vi "AI Post Step.vi"(8 "error in (no error)":errorcluster, 9 "AIRead":T1, 10 "Socket No":u16=1, 11 "NI Analog Input in":refnum<class "NI Analog Input.lvclass">) -> (0 "error out":errorcluster, 1 "AnalogRead":dbl[](array[numeric]), 2 "Report Text":string, 3 "NI Analog Input out":refnum<class "NI Analog Input.lvclass">, 4 "Selected Physical Channel":string[](array[string]))   [LabVIEW 2023, in "HardwareAbstractionLayer_LVOOP.lvlib" / "NI Analog Input.lvclass"]
uses:
  NI Analog Input.lvclass
  NI Analog Input.lvclass/NI Analog Input.ctl
  Database/Database.lvclass
  <resource>/objmgr/daqmx.rc
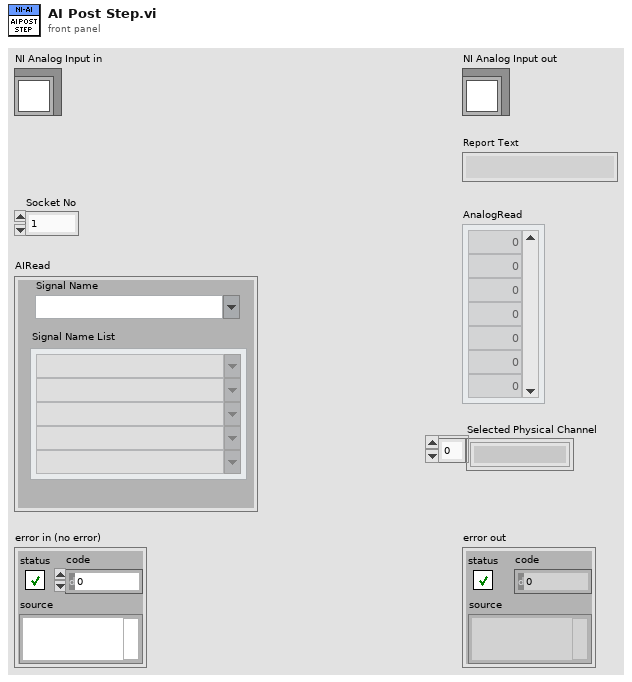
[diagram p1: front panel]
types:
  T1 = cluster{"Signal Name":string, "Signal Name List":string[]}
  T2 = cluster{"table":string, "condition":string, "columns":string[]}
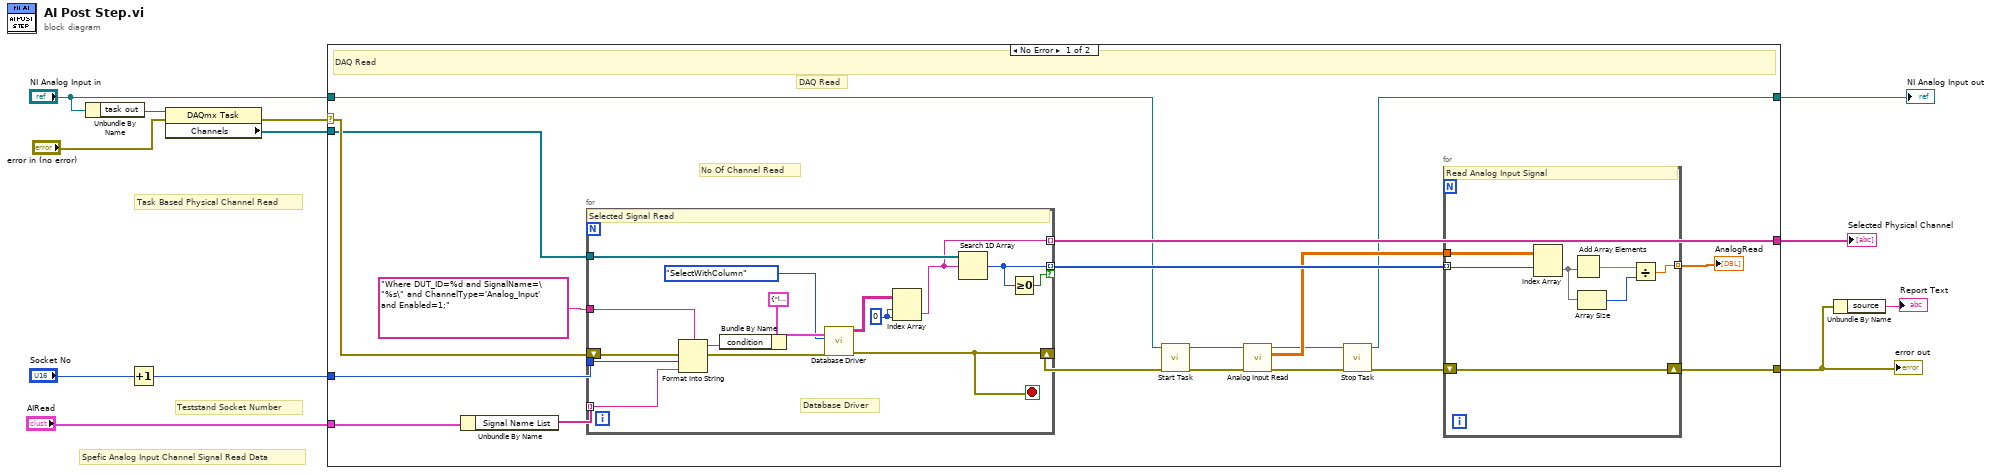
[diagram p0: block diagram]
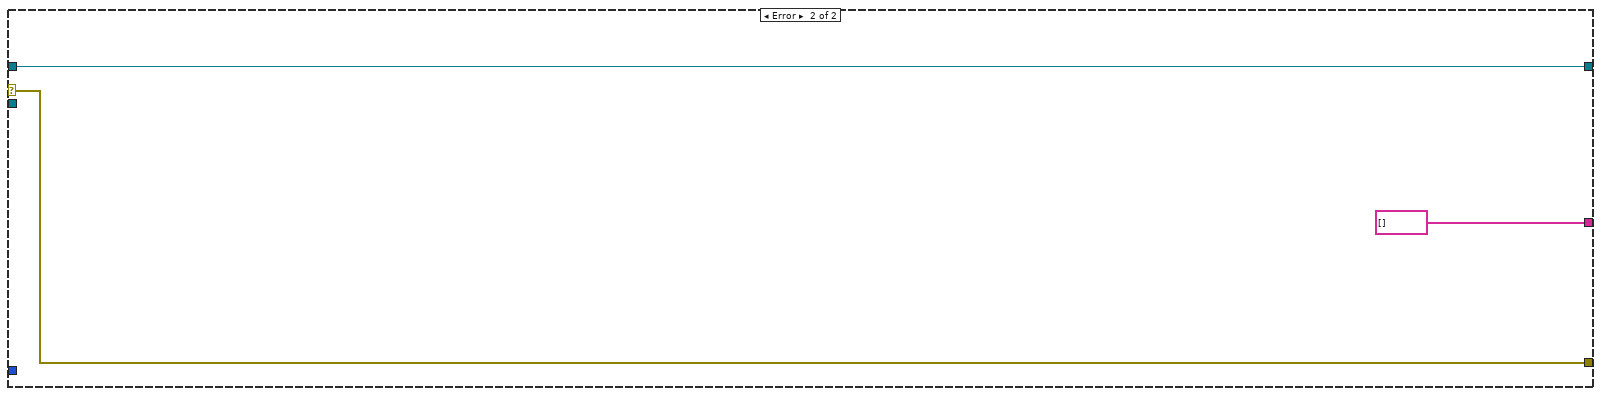
[diagram p2: hidden frame]
diagram:
  # "Teststand Socket Number"
  # "Spefic Analog Input Channel Signal Read Data"
  # "Task Based Physical Channel Read"
  n1 = Unbundle By Name("NI Analog Input in") -> ("task out"=w12:refnum<k21>)
  n2 = Increment(x="Socket No") -> (x+1=w4:u16)
  n3 = property class="DAQmx Task"(reference=w12, error in="error in (no error)") -> (error out=w2:errorcluster, "Channels"=w10:refnum<k21>[])  [unwired: 1 out]
  n4 = case shown="No Error" w2 {
    selector: w2 -> [w25 w56]
    tunnel: [w31 w56] -> w6
    tunnel: "AIRead" -> [w30 _]
    tunnel: w4 -> [w26 _]
    tunnel: w10 -> [w24 _]
    tunnel: "NI Analog Input in" -> [w20 w57]
    tunnel: [w15 w57] -> w7
    tunnel: [w21 string[] []] -> w1
    frame No Error {
      # "No Of Channel Read"
      # "DAQ Read"
      # "DAQ Read"
      n5 = Unbundle By Name(w30) -> ("Signal Name List"=w29:string[])
      n6 = for {
        tunnel: w29 -> [w45] mode=indexing
        tunnel: "Where DUT_ID=%d and SignalName=\"%s\" and ChannelType='Analog_Input' and Enabled=1;" -> [w47]
        tunnel: w26 -> [w46]
        shift-right: [w35] -> w18
        shift-left: w25 -> [w41]
        tunnel: [w37] -> w27 mode=indexing if=w36
        tunnel: w24 -> [w33]
        tunnel: [w32] -> w21 mode=indexing
        stop <- w35 stop-if-true
        w38 = 0 ("disabled index (col)")
        # "Database Driver"
        # "Selected Signal Read"
        n7 = Format Into String(format string=w47, error in=w41, w46, w45) -> (resulting string=w43:string, error out=w40:errorcluster)  [unwired: 1 in]
        n8 = Bundle By Name(cluster=T2 {"table"="ltt.daq_configuration", "condition"="Where ChannelType='Analog_Input' and Enabled=1", "columns"=["PhysicalChannel"]} ("SQLTableData"), "condition"=w43) -> (w42:T2)
        n9 = call "Database Driver.vi"("SQLTableData"=w42, "error in"=w40, "Select"=enum16{"SelectWithQuery", "SelectWithColumn"}."SelectWithColumn") -> ("error out"=w35:errorcluster, "data"=w39:string[][])  [unwired: 5 in, 2 out]
        n10 = Index Array(array=w39, index (row)=w38, index (col)=w38) -> (element=w32:string)
        n11 = Search 1D Array(1D array=w33, element=w32) -> (index of element=w37:i32)  [unwired: 1 in]
        n12 = Greater Or Equal To 0?(x=w37) -> (x >= 0?=w36:bool)
      }
      n13 = call-dynamic "Start Task.vi"("error in"=w18, "Analog Input in"=w20) -> ("error out"=w17:errorcluster, "Analog Input out"=w19:refnum<class "NI Analog Input.lvclass">)  [unwired: 8 in]
      n14 = call-dynamic "Analog Input Read.vi"("error in (no error)"=w17, "Analog Input in"=w19) -> ("error out"=w14:errorcluster, "data"=w22:dbl[][], "Analog Input out"=w16:refnum<class "NI Analog Input.lvclass">)  [unwired: 7 in]
      n15 = call-dynamic "Stop Task.vi"("error in"=w14, "Analog Input in"=w16) -> ("error out"=w13:errorcluster, "Analog Input out"=w15:refnum<class "NI Analog Input.lvclass">)  [unwired: 8 in]
      n16 = for {
        shift-right: [w54] -> w31
        shift-left: w13 -> [w54]
        tunnel: w22 -> [w53]
        tunnel: w27 -> [w52] mode=indexing
        tunnel: [w50] -> w23 mode=indexing
        # "Read Analog Input Signal"
        n17 = Index Array(array=w53, index (row)=w52) -> (element=w49:dbl[])  [unwired: 1 in]
        n18 = Add Array Elements(numeric array=w49) -> (sum=w51:dbl)
        n19 = Array Size(array=w49) -> (size(s)=w48:i32)
        n20 = Divide(x=w51, y=w48) -> (x/y=w50:dbl)
      }
      "AnalogRead" <- w23
    }
    frame Error {
    }
  }
  "error out" <- w6
  "NI Analog Input out" <- w7
  "Selected Physical Channel" <- w1
  n21 = Unbundle By Name(w6) -> ("source"=→"Report Text":string)
